vi "yolo_draw_results.vi"(6 "coco_names":path, 8 "error in (no error)":errorcluster, 10 "results":T2, 11 "image":refnum<class "Mat_8U.lvclass">) -> (0 "error out":errorcluster, 3 "img out":refnum<class "Mat_8U.lvclass">)   [LabVIEW 2023]
uses:
  <vilib>/addons/VIRobotics/opencv_yiku/Mat/Mat_8U/Mat_8U.lvclass
  <vilib>/addons/VIRobotics/opencv_yiku/ctls/Rect.ctl
  <vilib>/Utility/file.llb/Read Delimited Spreadsheet (string).vi
  <vilib>/addons/VIRobotics/opencv_yiku/opencv_yiku.lvlib
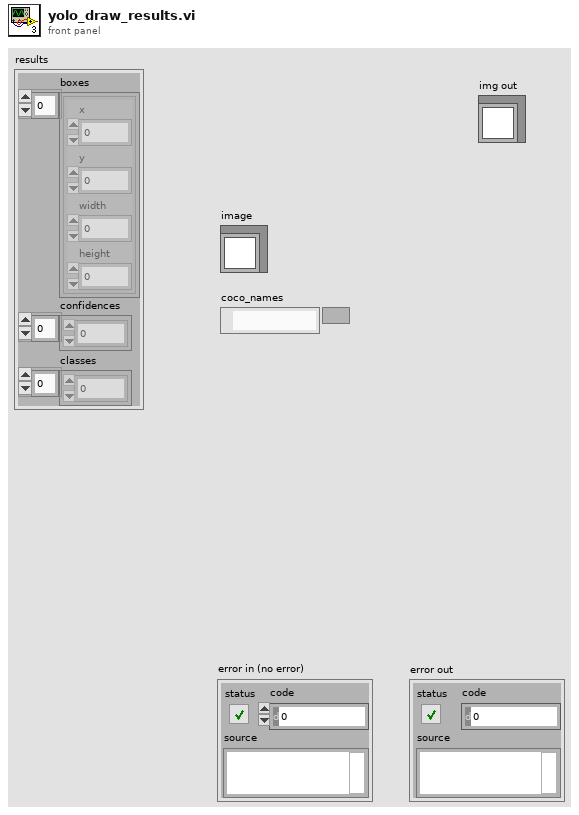
[diagram p1: front panel]
types:
  T1 = typedef "opencv_yiku.lvlib/Rect.ctl" = cluster{"x":i32, "y":i32, "width":i32, "height":i32}
  T2 = cluster{"boxes":T1[], "confidences":sgl[], "classes":i32[]}
  T3 = cluster{"Width":i16, "Style":enum32{"Solid", "Dash", "Dot", "DashDot", "DashDotDot"}}
  T4 = cluster{"Font Name:":string, "Size":i16, "Strikeout?":bool, "Italic?":bool, "Underline?":bool, "Outline?":bool, "Shadow?":bool, "Bold?":bool}
  T5 = enum16{"User-specified Font", "Application Font", "System Font", "Dialog Font"}
  T6 = cluster{"left":i16, "top":i16, "right":i16, "bottom":i16}
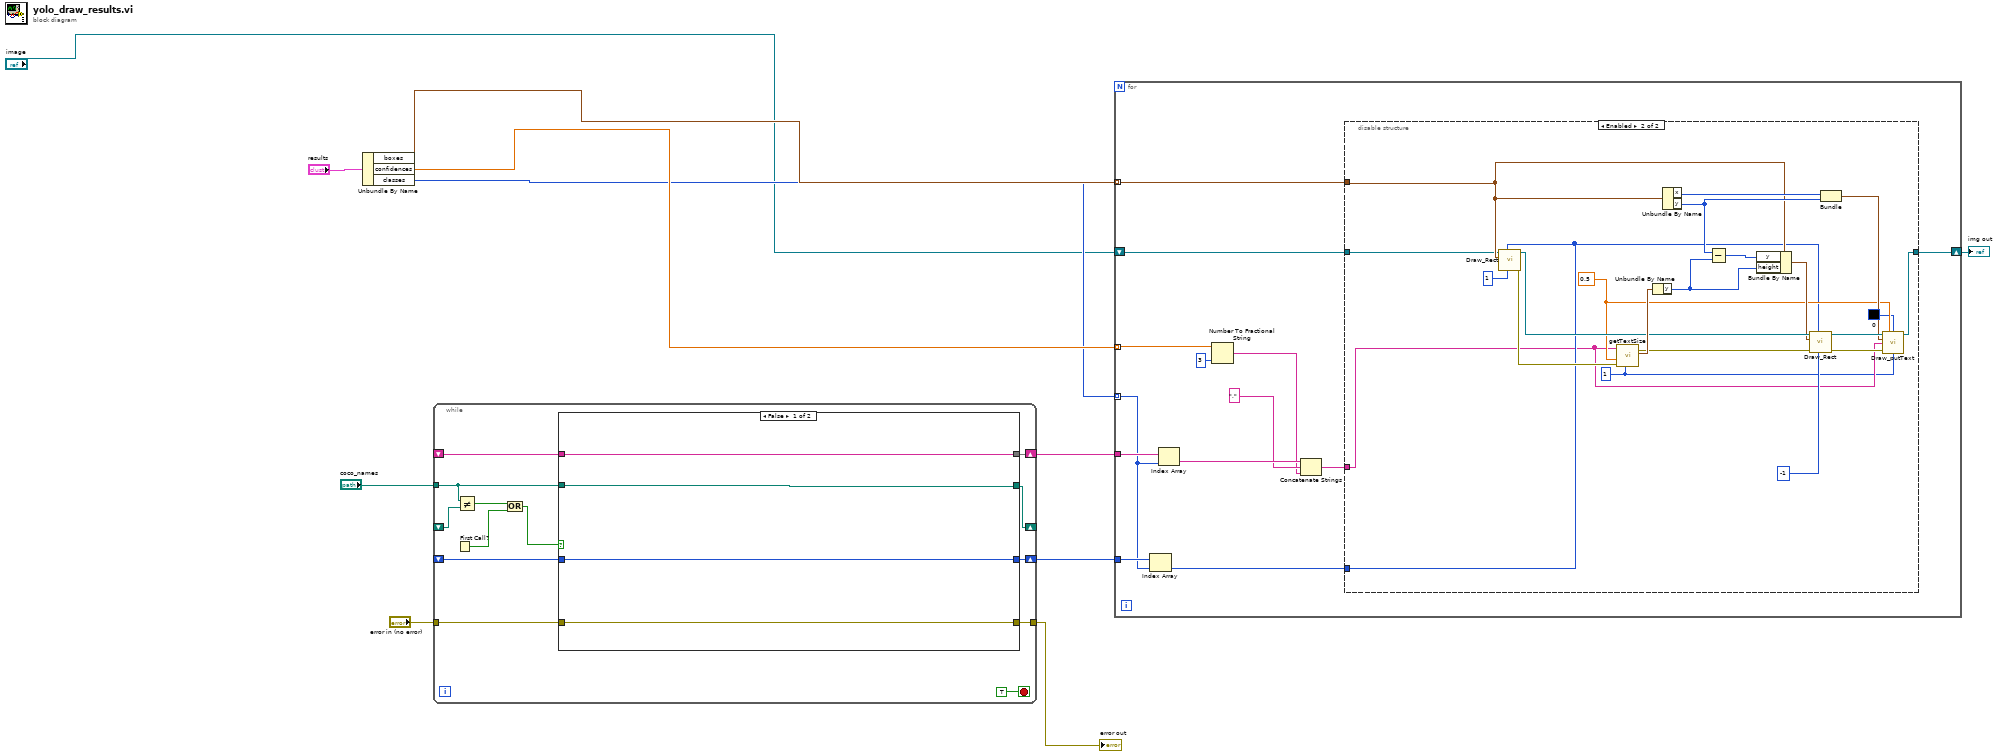
[diagram p0: block diagram]
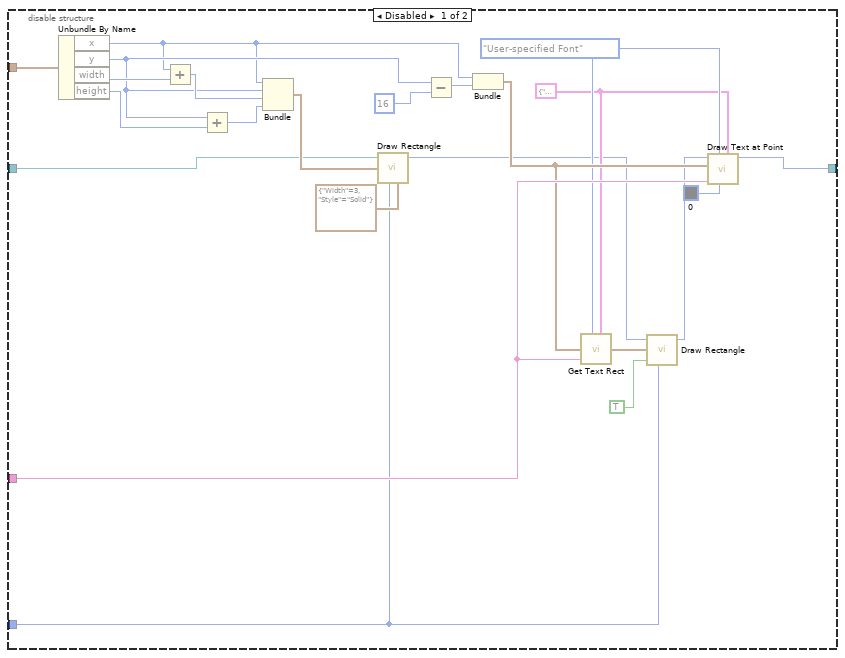
[diagram p2: hidden frame]
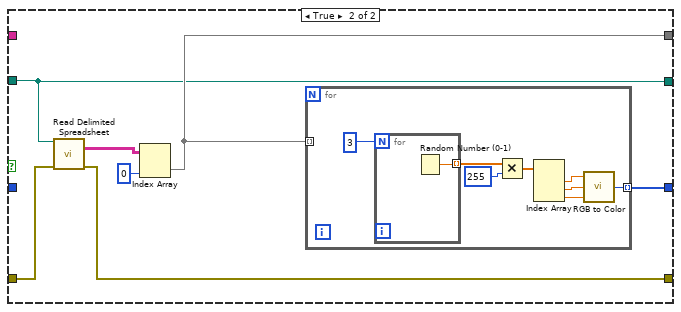
[diagram p3: hidden frame]
diagram:
  n1 = Unbundle By Name("results") -> ("boxes"=w6:T1[], "confidences"=w5:sgl[], "classes"=w4:i32[])
  n2 = while {
    shift-right: [w24] -> w11
    shift-left: _ -> [w21]
    shift-right: [w23] -> w10
    shift-left: _ -> [w20]
    tunnel: "error in (no error)" -> [w19]
    tunnel: [w18] -> w8
    shift-right: [w17] -> _
    shift-left: _ -> [w14]
    tunnel: "coco_names" -> [w15]
    stop <- TRUE stop-if-true
    n3 = First Call?() -> (First Call?: T/F=w16:bool)
    n4 = Not Equal?(x=w15, y=w14) -> (x != y?=w13:bool)
    n5 = Or(x=w13, y=w16) -> (x .or. y?=w12:bool)
    n6 = case shown="False" w12 {
      tunnel: [w28 w35] -> w24
      tunnel: [w27 w34] -> w23
      tunnel: w15 -> [w25 w29]
      tunnel: w21 -> [w28 _]
      tunnel: w20 -> [w27 _]
      tunnel: w19 -> [w26 w31]
      tunnel: [w26 w30] -> w18
      tunnel: [w25 w29] -> w17
      frame False {
      }
      frame True {
        n7 = call-poly <vilib>:"Read Delimited Spreadsheet.vi"("file path (dialog if empty)"=w29, "error in (no error)"=w31) -> ("all rows"=w32:string[][], "error out"=w30:errorcluster)  [unwired: 8 in, 4 out]
        n8 = Index Array(array=w32, index (col)=0 ("disabled index (col)")) -> (element=w35:string[])  [unwired: 1 in]
        n9 = for {
          tunnel: w35 -> [_] mode=indexing
          tunnel: [w36] -> w34 mode=indexing
          n10 = for {
            N: 3 -> [_]
            tunnel: [w44] -> w42 mode=indexing
            n11 = Random Number (0-1)() -> (number: 0 to 1=w44:dbl)
          }
          n12 = Multiply(x=w42, y=255) -> (x*y=w40:dbl[])
          n13 = Index Array(array=w40) -> (element #1=w39:dbl, element #2=w38:dbl, element #3=w37:dbl)  [unwired: 3 in]
          n14 = call <vilib>:"RGB to Color.vi"("B"=w37, "G"=w38, "R"=w39) -> ("Color"=w36:u32)
        }
      }
    }
  }
  "error out" <- w8
  n15 = for {
    tunnel: w6 -> [w56] mode=indexing
    tunnel: w4 -> [w49] mode=indexing
    tunnel: w5 -> [w52] mode=indexing
    tunnel: w10 -> [w57]
    tunnel: w11 -> [w55]
    shift-right: [w45] -> w1
    shift-left: "image" -> [w46]
    n16 = Index Array(array=w57, index=w49) -> (element=w47:u32)
    n17 = Index Array(array=w55, index=w49) -> (element=w54:string)
    n18 = Number To Fractional String(number=w52, precision (6)=i16 3) -> (F-format string=w50:string)  [unwired: 2 in]
    n19 = Concatenate Strings(w54, "," ("string"), w50) -> (w48:string)
    n20 = disable-structure shown="Enabled" {
      disable-tunnel: w56 -> [w80 w86]
      disable-tunnel: [w69 w82] -> w45
      disable-tunnel: w48 -> [w68 w83]
      disable-tunnel: w47 -> [w60 w85]
      disable-tunnel: w46 -> [w58 w84]
      frame Disabled {
        w65 = T4 {"Font Name:"="Times New Roman", "Size"=15, "Strikeout?"=FALSE, "Italic?"=FALSE, "Underline?"=FALSE, "Outline?"=FALSE, "Shadow?"=FALSE, "Bold?"=TRUE} ("[user-specified font]")
        w66 = T5."User-specified Font" ("desired font(Application)")
        n21 = Unbundle By Name(w80) -> ("x"=w70:i32, "y"=w73:i32, "width"=w79:i32, "height"=w78:i32)
        n22 = Add(x=w70, y=w79) -> (x+y=w77:i32)
        n23 = Add(x=w73, y=w78) -> (x+y=w76:i32)
        n24 = Bundle("x"=w70, "y"=w73, w77, w76) -> (w75:cluster{"x":i32, "y":i32, i32, i32})  [unwired: 1 in]
        n25 = call <vilib>:"Draw Rectangle.vi"("picture"=w58, "rect"=w75, "color(black)"=w60, "pen"=T3 {"Width"=3, "Style"=enum."Solid"}) -> ("new picture"=w64:picture)  [unwired: 5 in]
        n26 = Subtract(x=w73, y=16) -> (x-y=w71:i32)
        n27 = Bundle("x"=w70, w71) -> (w67:cluster{"x":i32, i32})  [unwired: 1 in]
        n28 = call <vilib>:"Get Text Rect.vi"("desired font(Application)"=w66, "origin(0,0)"=w67, "text"=w68, "[user-specified font]"=w65) -> ("rect"=w62:T6)  [unwired: 5 in]
        n29 = call <vilib>:"Draw Rectangle.vi"("picture"=w64, "rect"=w62, "fill?(F)"=TRUE, "color(black)"=w60) -> ("new picture"=w63:picture)  [unwired: 5 in]
        n30 = call <vilib>:"Draw Text at Point.vi"("[user-specified font]"=w65, "text color(black)"=u32 0, "desired font(Application)"=w66, "text"=w68, "origin"=w67, "picture"=w63) -> ("new picture"=w69:picture)  [unwired: 4 in, 1 out]
      }
      frame Enabled {
        w81 = 1 ("thickness")
        w92 = 0.5 ("fontScale")
        n31 = call <vilib>:"Draw_Rect.vi"("thickness"=1, "color"=w85, "rect"=w86, "Mat"=w84) -> ("error out"=w89:errorcluster, "Mat out"=w100:refnum<class "Mat_8U.lvclass">)  [unwired: 6 in]
        n32 = call <vilib>:"getTextSize.vi"("thickness"=w81, "error in (no error)"=w89, "fontScale"=w92, "text"=w83) -> ("error out"=w88:errorcluster, "size"=w101:cluster{"x":i32, "y":i32})  [unwired: 5 in, 1 out]
        n33 = Unbundle By Name(w101) -> ("y"=w97:i32)
        n34 = Unbundle By Name(w86) -> ("x"=w95:i32, "y"=w91:i32)
        n35 = Subtract(x=w91, y=w97) -> (x-y=w94:i32)
        n36 = Bundle By Name(cluster=w86, "y"=w94, "height"=w97) -> (w99:T1)
        n37 = call <vilib>:"Draw_Rect.vi"("thickness"=-1, "color"=w85, "error in (no error)"=w88, "rect"=w99, "Mat"=w100) -> ("error out"=w87:errorcluster, "Mat out"=w96:refnum<class "Mat_8U.lvclass">)  [unwired: 5 in]
        n38 = Bundle("x"=w95, "y"=w91) -> (w93:cluster{"x":i32, "y":i32})  [unwired: 1 in]
        n39 = call <vilib>:"Draw_putText.vi"("Mat"=w96, "fontScale"=w92, "color"=u32 0, "point"=w93, "text"=w83, "error in (no error)"=w87, "thickness"=w81) -> ("Mat out"=w82:refnum<class "Mat_8U.lvclass">)  [unwired: 7 in, 1 out]
      }
    }
  }
  "img out" <- w1
